vi "Complex selector (array of waveform CDB).vi"(10 "Domain (mag)":T1, 11 "Array of waveform (CDB)":waveform(cdb)[](array[waveform])) -> (3 "Part of array of waveform (DBL)":waveform(dbl)[](array[waveform]))   [LabVIEW 2020]
uses:
  Domain.ctl
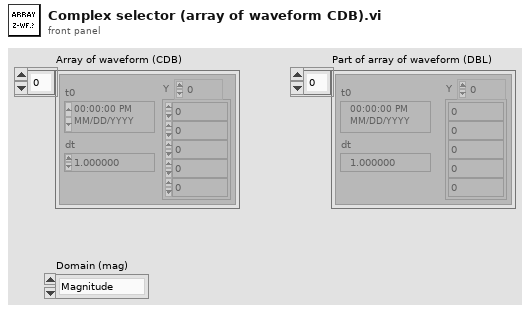
[diagram p1: front panel]
types:
  T1 = typedef "Domain.ctl" = enum16{"Magnitude", "Phase", "Phase unwrp", "Real", "Imaginary"}
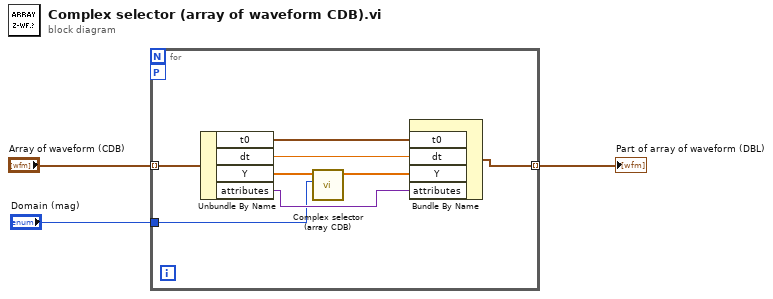
[diagram p0: block diagram]
diagram:
  n1 = for {
    tunnel: "Array of waveform (CDB)" -> [w11] mode=indexing
    tunnel: [w5] -> w2 mode=indexing
    workers-P: _ -> [_]
    tunnel: "Domain (mag)" -> [w4]
    n2 = Unbundle By Name(w11) -> ("t0"=w8:timestamp, "dt"=w7:dbl, "Y"=w10:cdb[], "attributes"=w6:variant)
    n3 = call "Complex selector (array CDB).vi"("Domain (mag)"=w4, "Array (CDB)"=w10) -> ("Part (DBL)"=w9:dbl[])  [unwired: 9 in]
    n4 = Bundle By Name("t0"=w8, "dt"=w7, "Y"=w9, "attributes"=w6) -> (w5:waveform(dbl))  [unwired: 1 in]
  }
  "Part of array of waveform (DBL)" <- w2
